vi "find peaks in ECG.vi"() -> ()   [LabVIEW 2017]
uses:
  <vilib>/Utility/file.llb/Read Delimited Spreadsheet (DBL).vi
  <vilib>/Analysis/Matrix/Numeric/Conversions/Array To Matrix - RA2.vi
  <vilib>/Analysis/Matrix/Numeric/Conversions/Matrix To Array - RM.vi
  <vilib>/Analysis/Matrix/NI_Matrix.lvlib
panel:
  out "appended array":dbl[][](array[numeric])
  out "XY Graph":cluster{dbl[], dbl[]}[](graph)
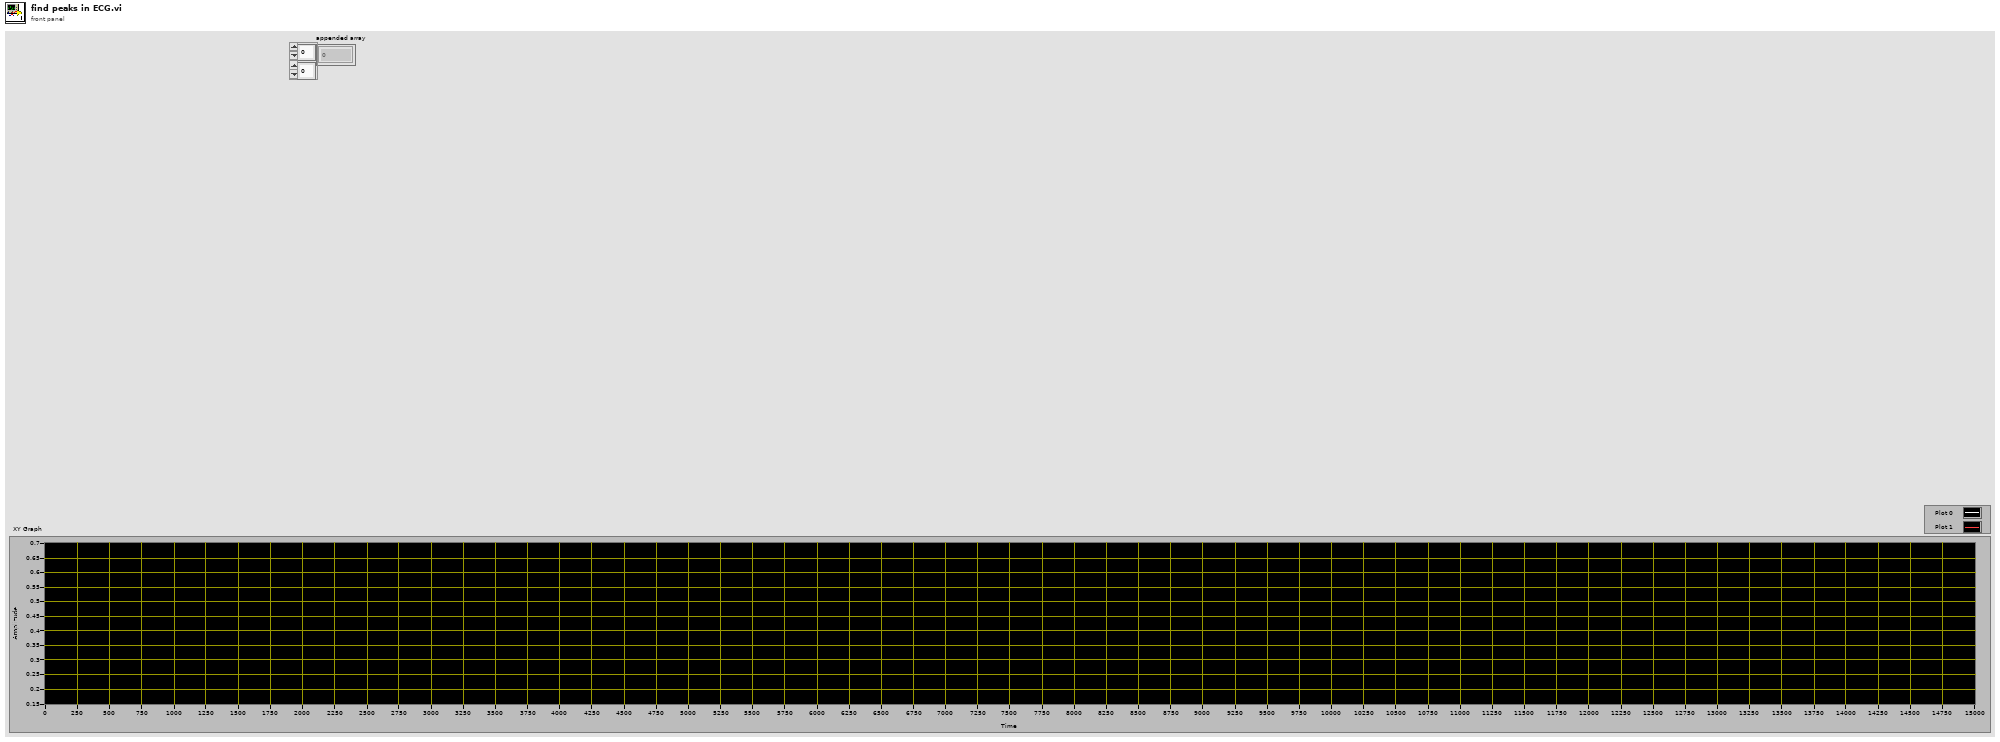
[diagram p1: front panel]
types:
  T1 = typedef "NI_Matrix.lvlib/RealMatrix.ctl" = dbl[][]
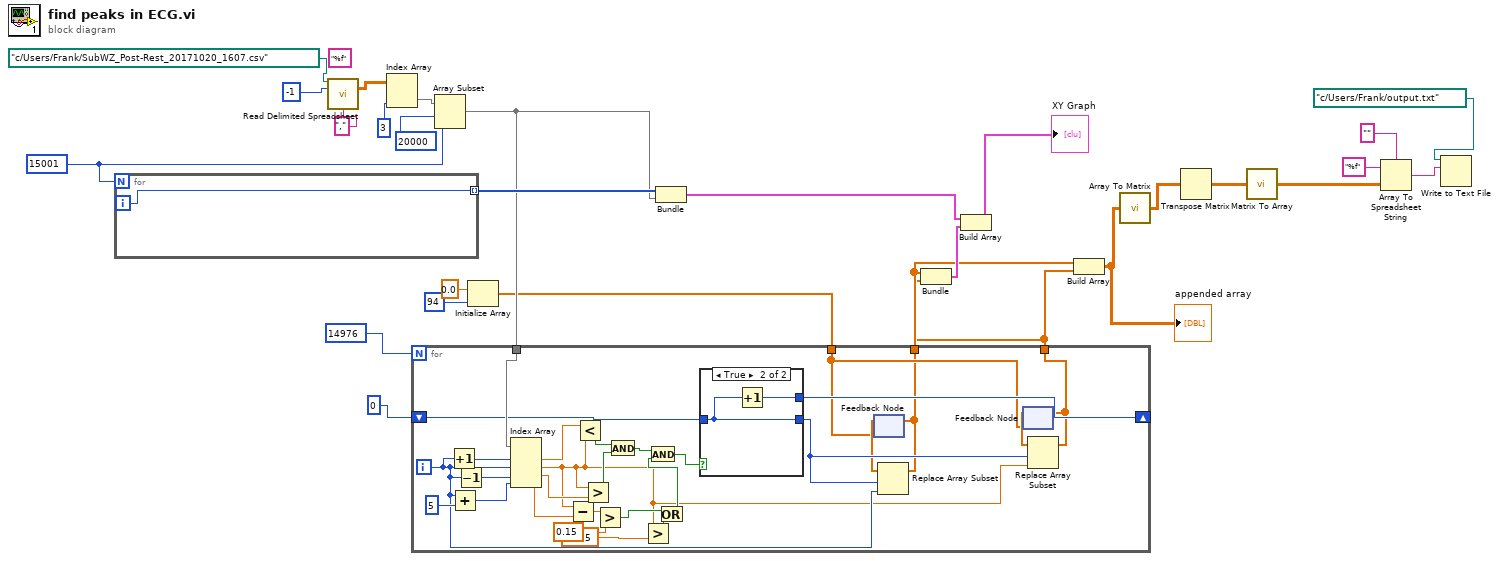
[diagram p0: block diagram]
diagram:
  w25 = 15001
  (unwired) "%f" ("format (%.3f)")
  n1 = for {
    N: w25 -> [_]
    tunnel: [w29] -> w20 mode=indexing
    i -> [w29]
  }
  n2 = call-poly <vilib>:"Read Delimited Spreadsheet.vi"("file path (dialog if empty)"=path "c:/Users/Frank/SubWZ_Post-Rest_20171020_1607.csv", "number of rows (all:-1)"=-1, "delimiter (\\t)"="," ("delimiter (\\t)")) -> ("all rows"=w15:dbl[][])  [unwired: 7 in, 5 out]
  n3 = Index Array(array=w15, index (col)=3 ("disabled index (col)")) -> (element=w27:dbl[])  [unwired: 1 in]
  n4 = Array Subset(array=w27, index=20000, length=w25) -> (w14:dbl[])
  n5 = Initialize Array(0.0 ("element"), 94 ("dimension size")) -> (w13:dbl[])
  n6 = for {
    N: 14976 -> [_]
    tunnel: w14 -> [w54]
    shift-right: [w57] -> _
    shift-left: 0 -> [w42]
    tunnel: [w38] -> w5
    tunnel: w13 -> [w36]
    tunnel: [w35] -> w6
    i -> [w41]
    n7 = Increment(x=w41) -> (x+1=w55:i32)
    n8 = Add(x=w41, y=5) -> (x+y=w50:i32)
    n9 = Decrement(x=w41) -> (x-1=w56:i32)
    n10 = Index Array(array=w54, index #1=w55, index #2=w41, index #3=w56, index #4=w50) -> (element #1=w53:dbl, element #2=w31:dbl, element #3=w52:dbl, element #4=w48:dbl)
    n11 = Subtract(x=w31, y=w48) -> (x-y=w47:dbl)
    n12 = Less?(x=w53, y=w31) -> (x < y?=w44:bool)
    n13 = Greater?(x=w31, y=w52) -> (0:w45:bool)
    n14 = Greater?(x=w47, y=0.15) -> (0:w33:bool)
    n15 = And(x=w44, y=w45) -> (x .and. y?=w43:bool)
    n16 = Greater?(x=w31, y=0.575) -> (0:w32:bool)
    n17 = Or(x=w33, y=w32) -> (x .or. y?=w34:bool)
    n18 = And(x=w43, y=w34) -> (x .and. y?=w51:bool)
    n19 = case shown="True" w51 {
      tunnel: [w58 w60] -> w57
      tunnel: w42 -> [w58 w59]
      tunnel: [w58 w59] -> w40
      frame False {
      }
      frame True {
        n20 = Increment(x=w59) -> (x+1=w60:i32)
      }
    }
    n21 = feedback #1(w36) -> (w37:dbl[])
    n22 = Replace Array Subset(array=w37, new element=w41, index=w40) -> (w35:dbl[])
    n23 = feedback-in #1(w35) -> ()
    n24 = feedback #2(w36) -> (w39:dbl[])
    n25 = Replace Array Subset(array=w39, new element=w31, index=w40) -> (w38:dbl[])
    n26 = feedback-in #2(w38) -> ()
  }
  n27 = Bundle(w20, w14) -> (w19:cluster{i32[], dbl[]})  [unwired: 1 in]
  n28 = Bundle(w6, w5) -> (w12:cluster{dbl[], dbl[]})  [unwired: 1 in]
  n29 = Build Array(w19, w12) -> (→"XY Graph":cluster{dbl[], dbl[]}[])
  n30 = Build Array(w6, w5) -> (w4:dbl[][])
  "appended array" <- w4
  n31 = call-poly <vilib>:"Array To Matrix.vi"("Real 2D Array"=w4) -> ("Real Matrix"=w3:T1)
  n32 = Transpose Matrix(1:w3) -> (0:w2:T1)
  n33 = call-poly <vilib>:"Matrix To Array.vi"("Real Matrix"=w2) -> ("Real 2D Array"=w1:dbl[][])
  n34 = Array To Spreadsheet String(delimiter (Tab)="", array=w1, 3:"%f" ("format string")) -> (spreadsheet string=w10:string)
  n35 = Write to Text File(file (use dialog)=path "c:/Users/Frank/output.txt" ("file path (dialog if empty)"), text=w10) -> ()  [unwired: 2 in, 3 out]
